vi "Set Property Method.vi"(10 "Theme Choice":T2, 11 "Cluster":T1) -> (3 "Cluster Out":T1)   [LabVIEW 2019, in "LSS.lvlib"]
doc: "Sets the style of front panel objects using property nodes.\n\n<b>Inputs:</b>\n<b>Cluster</b> - Cluster of all front panel objects.\n<b>Theme Choice</b> - Select theme to apply to front panel objects.\n\n<b>Outputs:</b>\n<b>Cluster out</b> - duplicate"
uses:
  LSS.lvlib
  Before UI References.ctl
  Themes.ctl
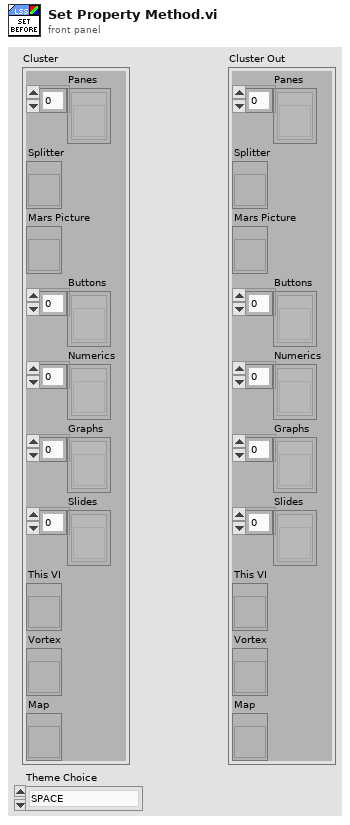
[diagram p1: front panel]
types:
  T1 = typedef "LSS.lvlib/Before UI References.ctl" = cluster{"Panes":refnum<vi>[], "Splitter":refnum<vi>, "Mars Picture":refnum<vi>, "Buttons":refnum<vi>[], "Numerics":refnum<vi>[], "Graphs":refnum<vi>[], "Slides":refnum<vi>[], "This VI":refnum<vi>, "Vortex":refnum<vi>, "Map":refnum<vi>}
  T2 = typedef "LSS.lvlib/Themes.ctl" = enum16{"SPACE", "ATK", "THEME1", "THEME2"}
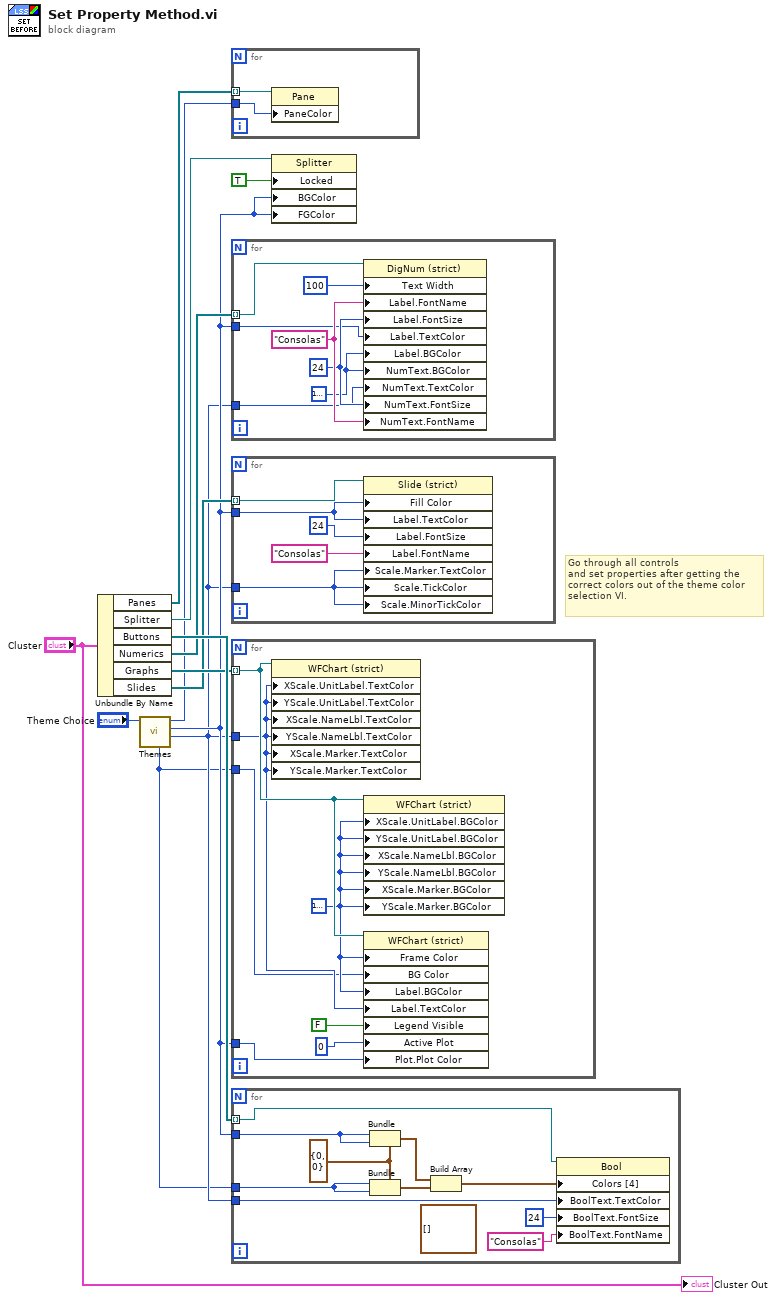
[diagram p0: block diagram]
diagram:
  # "Go through all controls\nand set properties after getting the\ncorrect colors out of the theme color\nselection VI."
  n1 = Unbundle By Name("Cluster") -> ("Panes"=w12:refnum<vi>[], "Splitter"=w13:refnum<vi>, "Buttons"=w9:refnum<vi>[], "Numerics"=w8:refnum<vi>[], "Graphs"=w7:refnum<vi>[], "Slides"=w6:refnum<vi>[])
  n2 = call "Themes.vi"("Theme Choice"="Theme Choice") -> ("Text"=w2:u32, "Accent"=w4:u32, "BG Color"=w3:u32, "Accent2"=w1:u32)  [unwired: 7 in]
  n3 = for {
    tunnel: w12 -> [w15] mode=indexing
    tunnel: w3 -> [w14]
    n4 = property on="Property Node" class="Pane"(reference=w15, "PaneColor"=w14) -> ()  [unwired: 1 in, 2 out]
  }
  n5 = for {
    tunnel: w8 -> [w22] mode=indexing
    tunnel: w4 -> [w17]
    tunnel: w2 -> [w16]
    w18 = u32 16777216
    w21 = "Consolas" ("Boolean Text.Font:Name")
    w20 = u32 24 ("Boolean Text.Font:Size")
    n6 = property class="DigNum (strict)"(reference=w22, "Text Width"=u32 100, "Label.FontName"=w21, "Label.FontSize"=w20, "Label.TextColor"=w17, "Label.BGColor"=w18, "NumText.BGColor"=w18, "NumText.TextColor"=w16, "NumText.FontSize"=w20, "NumText.FontName"=w21) -> ()  [unwired: 1 in, 2 out]
  }
  n7 = for {
    tunnel: w6 -> [w27] mode=indexing
    tunnel: w4 -> [w24]
    tunnel: w2 -> [w23]
    n8 = property class="Slide (strict)"(reference=w27, "Fill Color"=w24, "Label.TextColor"=w24, "Label.FontSize"=u32 24 ("Boolean Text.Font:Size"), "Label.FontName"="Consolas" ("Boolean Text.Font:Name"), "Scale.Marker.TextColor"=w23, "Scale.TickColor"=w23, "Scale.MinorTickColor"=w23) -> ()  [unwired: 1 in, 2 out]
  }
  n9 = for {
    tunnel: w7 -> [w34] mode=indexing
    tunnel: w4 -> [w30]
    tunnel: w2 -> [w29]
    tunnel: w1 -> [w28]
    w33 = u32 16777216
    n10 = property class="WFChart (strict)"(reference=w34, "XScale.UnitLabel.TextColor"=w29, "YScale.UnitLabel.TextColor"=w29, "XScale.NameLbl.TextColor"=w29, "YScale.NameLbl.TextColor"=w29, "XScale.Marker.TextColor"=w29, "YScale.Marker.TextColor"=w29) -> ()  [unwired: 1 in, 2 out]
    n11 = property class="WFChart (strict)"(reference=w34, "XScale.UnitLabel.BGColor"=w33, "YScale.UnitLabel.BGColor"=w33, "XScale.NameLbl.BGColor"=w33, "YScale.NameLbl.BGColor"=w33, "XScale.Marker.BGColor"=w33, "YScale.Marker.BGColor"=w33) -> ()  [unwired: 1 in, 2 out]
    n12 = property class="WFChart (strict)"(reference=w34, "Frame Color"=w33, "BG Color"=w28, "Label.BGColor"=w33, "Label.TextColor"=w29, "Legend Visible"=FALSE ("Legend:Visible"), "Active Plot"=u32 0, "Plot.Plot Color"=w30) -> ()  [unwired: 1 in, 2 out]
  }
  n13 = for {
    tunnel: w9 -> [w44] mode=indexing
    tunnel: w4 -> [w37]
    tunnel: w2 -> [w36]
    tunnel: w1 -> [w35]
    w43 = cluster{u32, u32} {0, 0}
    (unwired) cluster{u32, u32}[] [] ("Colors [4]")
    n14 = Bundle(cluster=w43, w37, w37) -> (w42:cluster{u32, u32})
    n15 = Bundle(cluster=w43, w35, w35) -> (w41:cluster{u32, u32})
    n16 = Build Array(w42, w41) -> (w40:cluster{u32, u32}[])
    n17 = property on="Property Node" class="Bool"(reference=w44, "Colors [4]"=w40, "BoolText.TextColor"=w36, "BoolText.FontSize"=u32 24 ("Boolean Text.Font:Size"), "BoolText.FontName"="Consolas" ("Boolean Text.Font:Name")) -> ()  [unwired: 1 in, 2 out]
  }
  n18 = property on="Property Node" class="Splitter"(reference=w13, "Locked"=TRUE ("Splitter Position Locked"), "BGColor"=w4, "FGColor"=w4) -> ()  [unwired: 1 in, 2 out]
  "Cluster Out" <- "Cluster"
